vi "FGZ_Stoper.vi"(4 "StoperEnum":T1) -> (1 "time (s)":dbl)   [LabVIEW 2024]
uses:
  StoperEnum.ctl
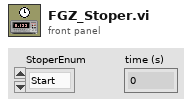
[diagram p1: front panel]
types:
  T1 = typedef "StoperEnum.ctl" = enum16{"Start", "Time"}
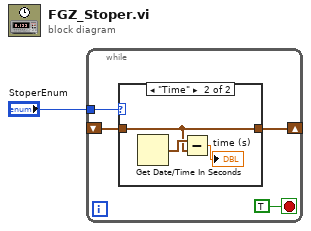
[diagram p0: block diagram]
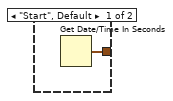
[diagram p2: hidden frame]
diagram:
  n1 = while {
    shift-right: [w3] -> _
    shift-left: _ -> [w2]
    tunnel: "StoperEnum" -> [w4]
    stop <- TRUE stop-if-true
    n2 = case shown="\"Time\"" w4 {
      tunnel: [w6 w7] -> w3
      tunnel: w2 -> [_ w7]
      frame "Start", Default {
        n3 = Get Date/Time In Seconds() -> (seconds since 1Jan1904=w6:timestamp)
      }
      frame "Time" {
        n4 = Get Date/Time In Seconds() -> (seconds since 1Jan1904=w8:timestamp)
        n5 = Subtract(x=w8, y=w7) -> (x-y=→"time (s)":dbl)
      }
    }
  }
